vi "Picture Selection.vi"() -> (2 "Valve Pictures":T1={"Command"={"Error"=enum."InError", "Config"=enum."InConfig", "Stale"=enum."InStale", "Close"=enum."InClose", "Open"=enum."InOpen", "TranClose"=enum."Blank", "TranOpen"=enum."Blank"}, "Feedback"={"Error"=enum."OutError", "Config"=enum."OutConfig", "Stale"=enum."OutStale", "Closed"=enum."OutClose", "Open"=enum."OutOpen", "TranClose"=enum."OutTranClose", "TranOpen"=enum."Blank"}, "Energized"={"Error"=enum."EnError", "Config"=enum."EnConfig", "Stale"=enum."EnStale", "False"=enum."EnOff", "True"=enum."EnOn"}})   [LabVIEW 2020, in "VolatusGUIElements.lvlib" / "2WayValveH.lvclass"]
uses:
  2WayValveH.lvclass
  Valve Pictures.ctl
  Command Pictures.ctl
  Picture.ctl
  Feedback Pictures.ctl
  Energized Pictures.ctl
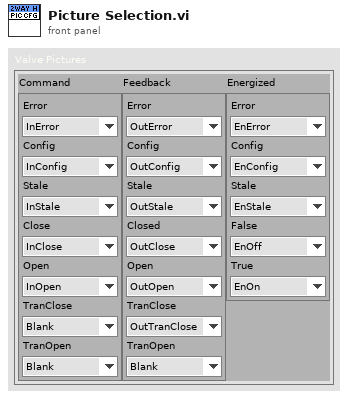
[diagram p1: front panel]
types:
  T1 = typedef "VolatusGUIElements.lvlib/2WayValveH.lvclass/Valve Pictures.ctl" = cluster{"Command":T2, "Feedback":T4, "Energized":T5}
  T2 = typedef "VolatusGUIElements.lvlib/2WayValveH.lvclass/Command Pictures.ctl" = cluster{"Error":T3, "Config":T3, "Stale":T3, "Close":T3, "Open":T3, "TranClose":T3, "TranOpen":T3}
  T3 = typedef "VolatusGUIElements.lvlib/2WayValveH.lvclass/Picture.ctl" = enum16{"Blank", "OutClose", "OutOpen", "OutTranClose", "OutTranOpen", "OutConfig", "OutStale", "OutError", "InClose", "InOpen", "InTranClose", "InTranOpen", "InConfig", "InStale", "InError", "EnOff", "EnOn", "EnConfig", "EnStale", "EnError"}
  T4 = typedef "VolatusGUIElements.lvlib/2WayValveH.lvclass/Feedback Pictures.ctl" = cluster{"Error":T3, "Config":T3, "Stale":T3, "Closed":T3, "Open":T3, "TranClose":T3, "TranOpen":T3}
  T5 = typedef "VolatusGUIElements.lvlib/2WayValveH.lvclass/Energized Pictures.ctl" = cluster{"Error":T3, "Config":T3, "Stale":T3, "False":T3, "True":T3}
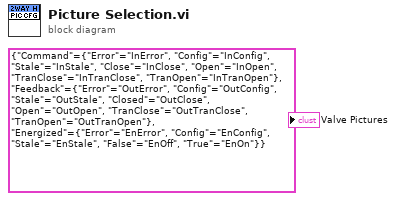
[diagram p0: block diagram]
diagram:
  "Valve Pictures" <- T1 {"Command"={"Error"=enum."InError", "Config"=enum."InConfig", "Stale"=enum."InStale", "Close"=enum."InClose", "Open"=enum."InOpen", "TranClose"=enum."InTranClose", "TranOpen"=enum."InTranOpen"}, "Feedback"={"Error"=enum."OutError", "Config"=enum."OutConfig", "Stale"=enum."OutStale", "Closed"=enum."OutClose", "Open"=enum."OutOpen", "TranClose"=enum."OutTranClose", "TranOpen"=enum."OutTranOpen"}, "Energized"={"Error"=enum."EnError", "Config"=enum."EnConfig", "Stale"=enum."EnStale", "False"=enum."EnOff", "True"=enum."EnOn"}} ("Valve Pictures")
